vi "Handle Command.vi"(8 "error in (no error)":errorcluster, 9 "Data":variant, 10 "Command":string, 11 "Instrument.SR7270 in":refnum<class "Instrument.SR7270.lvclass">) -> (0 "error out":errorcluster, 1 "Processed Data":variant, 2 "Command":string, 3 "Instrument.SR7270 out":refnum<class "Instrument.SR7270.lvclass">)   [LabVIEW 2016, in "Instrument.SR7270.lvclass"]
uses:
  Instrument.SR7270.lvclass
  Typedefs/SignalChannelConfig--Cluster.ctl
  Driver/Typedefs/VMODE--enum.ctl
  Driver/Typedefs/FLOAT--enum.ctl
  Driver/Typedefs/FET--enum.ctl
  Driver/Typedefs/LF--enum.ctl
  Instrument.SR7270.lvclass/Instrument.SR7270.ctl
  Driver/Typedefs/SEN-IMODE0--enum.ctl
  levylab_inst/lvsrc/SMOs/Instrument/Instrument.lvclass
  Driver/SR7270 Drivers.lvclass
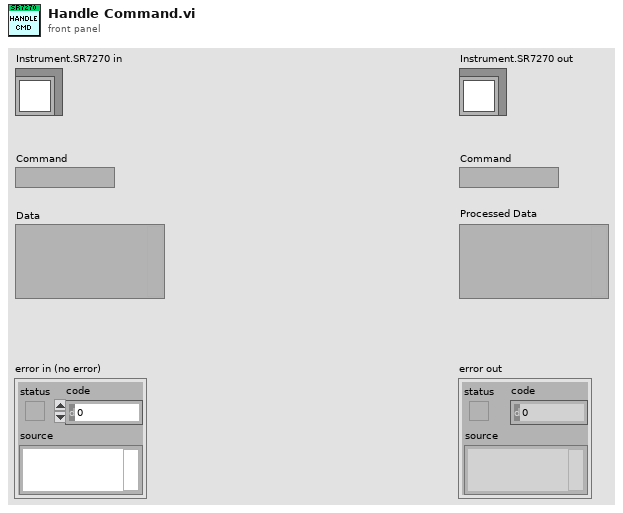
[diagram p1: front panel]
types:
  T1 = typedef "Instrument.SR7270.lvclass/SignalChannelConfig--Cluster.ctl" = cluster{"Input Mode":T2, "Input Connector Shell":T3, "Input Device":T4, "Line Rejection Filter":T5}
  T2 = typedef "SR7270 Drivers.lvclass/VMODE--enum.ctl" = enum16{"Both Grounded", "A input only", "-B input only", "A-B differential"}
  T3 = typedef "SR7270 Drivers.lvclass/FLOAT--enum.ctl" = enum16{"Ground", "Float"}
  T4 = typedef "SR7270 Drivers.lvclass/FET--enum.ctl" = enum16{"Bipolar", "FET"}
  T5 = typedef "SR7270 Drivers.lvclass/LF--enum.ctl" = enum16{"Off", "60 Hz", "120 Hz", "60 & 120 Hz"}
  T6 = typedef "SR7270 Drivers.lvclass/SEN-IMODE0--enum.ctl" = enum16{"2 nV", "5 nV", "10 nV", "20 nV", "50 nV", "100 nV", "200 nV", "500 nV", "1 µV", "2 µV", "5 µV", "10 µV", "20 µV", "50 µV", "100 µV", "200 µV", "500 µV", "1 mV", "2 mV", "5 mV", "10 mV", "20 mV", "50 mV", "100 mV", "200 mV", "500 mV", "1 V"}
  T7 = typedef "Instrument.SR7270.lvclass/getAll.ctl" = cluster{"X (V or A)":dbl, "Y (V or A)":dbl, "Mag (V or A)":dbl, "Phase (°)":dbl, "Oscillator Amplitude (V)":dbl, "Oscillator frequency (Hz)":dbl, "REF time constant (s)":dbl, "REF harmonic":u16, "REF phase (°)":dbl, "REF frequency (Hz)":dbl, "AC Gain":string, "Current Mode":string, "AC-DC Coupling":string, "FET":string, "Float":string, "Line Filter":string, "Voltage Mode":string, "Sensitivty (V or A)":dbl}
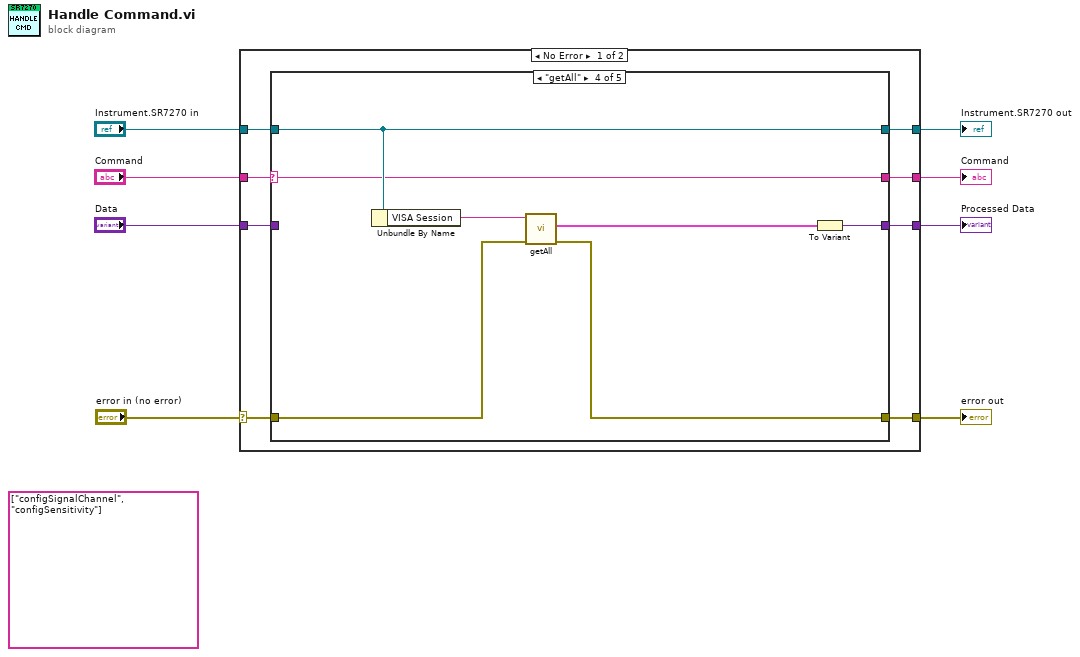
[diagram p0: block diagram]
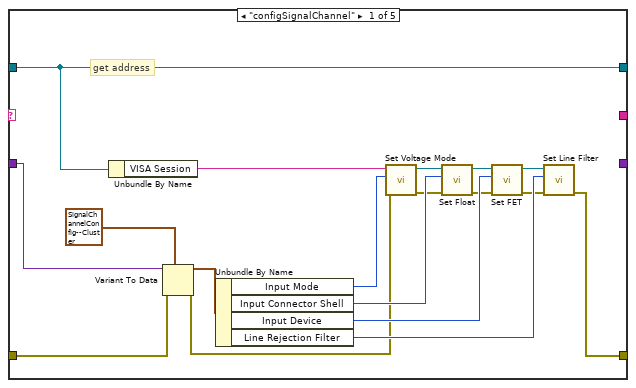
[diagram p2: hidden frame]
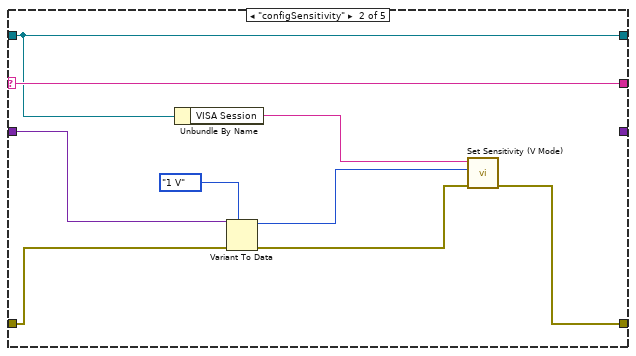
[diagram p3: hidden frame]
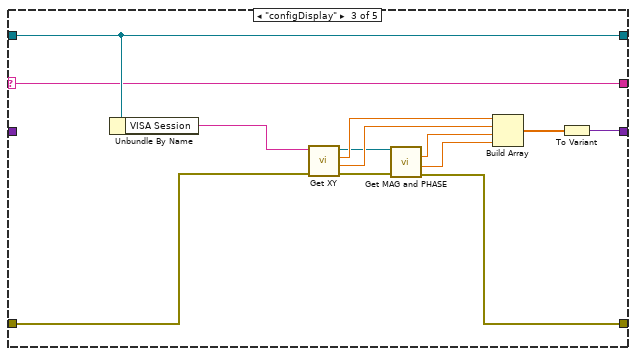
[diagram p4: hidden frame]
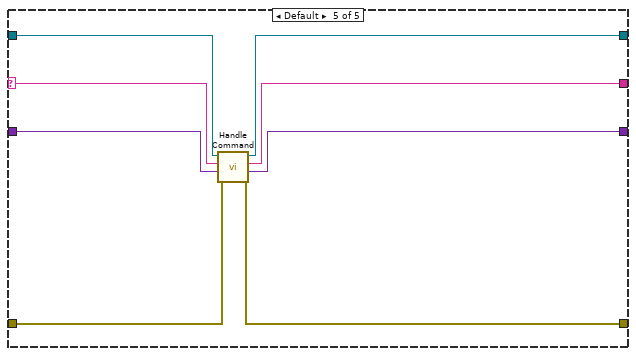
[diagram p5: hidden frame]
diagram:
  (unwired) string[] ["configSignalChannel", "configSensitivity"] ("element")
  n1 = case shown="No Error" "error in (no error)" {
    selector: "error in (no error)" -> [w11 w72]
    tunnel: [w10 w72] -> w8
    tunnel: [w16 _] -> w7
    tunnel: [w15 _] -> w6
    tunnel: [w14 w73] -> w5
    tunnel: "Data" -> [w13 _]
    tunnel: "Command" -> [w9 _]
    tunnel: "Instrument.SR7270 in" -> [w12 w73]
    frame No Error {
      n2 = case shown="\"getAll\"" w9 {
        selector: w9 -> [_ w43 w55 w62 w64]
        tunnel: [_ _ w54 w61 w71] -> w16
        tunnel: [_ w43 w55 w62 w70] -> w15
        tunnel: [w33 w42 w56 w63 w69] -> w14
        tunnel: w13 -> [w34 w40 _ _ w68]
        tunnel: w12 -> [w33 w42 w56 w63 w67]
        tunnel: w11 -> [w32 w41 w52 w59 w66]
        tunnel: [w18 w37 w50 w58 w65] -> w10
        frame "configSignalChannel" {
          # "get address"
          n3 = Unbundle By Name(w33) -> ("VISA Session"=w30:string)
          n4 = Variant To Data(error in=w32, type=T1 {"Input Mode"=enum."A input only", "Input Connector Shell"=enum."Float", "Input Device"=enum."Bipolar", "Line Rejection Filter"=enum."Off"} ("Signal Channel Config"), Variant=w34) -> (data=w29:T1, error out=w17:errorcluster)
          n5 = Unbundle By Name(w29) -> ("Input Mode"=w28:T2, "Input Connector Shell"=w26:T3, "Input Device"=w27:T4, "Line Rejection Filter"=w25:T5)
          n6 = call "Set Voltage Mode.vi"("error in (no error)"=w17, "Voltage Mode"=w28, "VISA resource name"=w30) -> ("error out"=w23:errorcluster, "VISA resource name out"=w24:refnum<visa-resource-name>)  [unwired: 7 in]
          n7 = call "Set Float.vi"("error in (no error)"=w23, "Float Mode"=w26, "VISA resource name"=w24) -> ("error out"=w21:errorcluster, "VISA resource name out"=w22:refnum<visa-resource-name>)  [unwired: 7 in]
          n8 = call "Set FET.vi"("error in (no error)"=w21, "FET Mode"=w27, "VISA resource name"=w22) -> ("error out"=w19:errorcluster, "VISA resource name out"=w20:refnum<visa-resource-name>)  [unwired: 7 in]
          n9 = call "Set Line Filter.vi"("error in (no error)"=w19, "Line Frequency Rejection"=w25, "VISA resource name"=w20) -> ("error out"=w18:errorcluster)  [unwired: 7 in, 1 out]
        }
        frame "configSensitivity" {
          n10 = Unbundle By Name(w42) -> ("VISA Session"=w35:string)
          n11 = Variant To Data(error in=w41, type=SEN-IMODE0--enum."1 V" ("Sensitivity IMODE0"), Variant=w40) -> (data=w39:T6, error out=w38:errorcluster)
          n12 = call "Set Sensitivity (V Mode).vi"("error in (no error)"=w38, "Sensitivity IMODE0"=w39, "VISA resource name"=w35) -> ("error out"=w37:errorcluster)  [unwired: 7 in, 1 out]
        }
        frame "configDisplay" {
          n13 = Unbundle By Name(w56) -> ("VISA Session"=w53:string)
          n14 = call "Get XY.vi"("error in (no error)"=w52, "VISA resource name"=w53) -> ("error out"=w51:errorcluster, "Y (V or A)"=w48:dbl, "X (V or A)"=w49:dbl, "VISA resource name out"=w44:refnum<visa-resource-name>)  [unwired: 6 in]
          n15 = call "Get MAG and PHASE.vi"("error in (no error)"=w51, "VISA resource name"=w44) -> ("error out"=w50:errorcluster, "Phase (°)"=w46:dbl, "Magnitude (V or A)"=w47:dbl)  [unwired: 6 in, 1 out]
          n16 = Build Array(w49, w48, w47, w46) -> (w45:dbl[])
          n17 = To Variant(anything=w45) -> (Variant=w54:variant)
        }
        frame "getAll" {
          n18 = Unbundle By Name(w63) -> ("VISA Session"=w60:string)
          n19 = call "getAll.vi"("error in (no error)"=w59, "VISA Session"=w60) -> ("error out"=w58:errorcluster, "SR7270 getAll"=w57:T7)  [unwired: 7 in, 1 out]
          n20 = To Variant(anything=w57) -> (Variant=w61:variant)
        }
        frame Default {
          n21 = call-parent "Handle Command.vi"("error in (no error)"=w66, "Data"=w68, "Command"=w64, "Instrument in"=w67) -> ("error out"=w65:errorcluster, "Processed Data"=w71:variant, "Command"=w70:string, "Instrument out"=w69:refnum<class "Instrument.SR7270.lvclass">)  [unwired: 4 in]
        }
      }
    }
    frame Error {
    }
  }
  "error out" <- w8
  "Instrument.SR7270 out" <- w5
  "Processed Data" <- w7
  "Command" <- w6
